vi "AcquireSingleScan.vi"() -> ()   [LabVIEW 2024]
uses:
  X-Scales.ctl
  ff6a1ae8-2aae-4c4f-bccd-18872fa50bd4.vi
  Program Files (x86)/Luna Technologies/OVA 5000 v5.14.2/data/OVA32.dll
panel:
  in  "Num Averages":u32=1
  in  "Output Spreadsheet File Path":path=path "C:/ss.txt"
  in  "Source Matrix":u8(ring) items=["A", "B", "C"]
  in  "Graph Data to Output":bool[](array[boolean])
  in  "Filter?":bool=TRUE
  in  "Resolution BW (GHz)":dbl=5.0 format="%.2f"
  in  "RBW Units for Output":u8(ring) items=["pm", "GHz"]
  in  "Cursor Indices":u32[](array[numeric])=[0, 0]
  in  "Device Descriptor":string
  in  "chanwidthstr":string
  out "error out":errorcluster
  in  "error in (no error)":errorcluster
  in  "Save Data":bool
  in  "Plot Data":bool
  in  "New Scan":bool
  out "Finding DUT Length":bool
  in  "Find DUT Length?":bool
  in  "filter data?":bool
  out "Graph":T1(graph) caption="Insertion Loss"
  in  "X-axis units":T2
  in  "Group Index":dbl=1.5 format="%.2f"
  in  "res BW (GHz)":dbl format="%.2f"
  out "genOutput":dbl[](array[numeric]) format="%.2f"
  in  "Graph Sel":u16(ring) items=["Insertion Loss", "Group Delay", "Chromatic Dispersion", "Polarization Dependent Loss", "Polarization Mode Dispersion", "Linear Phase Deviation", "Quadratic Phase Deviation", "Jones Matrix Element Amplitudes", "Jones Matrix Element Phases", "Time Domain Amplitude", "Time Domain Wavelength", "Min/Max Loss", "Second Order PMD", "Phase Ripple Linear", "Phase Ripple Quadratic"]
  out "error":errorcluster
  in  "Length of DUT (m)":dbl=3.0 format="%.3f"
  in  "Center WL":dbl=1550.0 caption="Center Wavelength (nm)" step=0.01 format="%.2f"
  in  "Meas Type":u16(ring)=1 caption="Type of Measurement" items=["Reflection", "Transmission"]
  in  "WL Range":u16(ring)=2 caption="Wavelength Range (nm)" items=["0.63", "1.27", "2.54", "5.09", "10.22", "20.58", "41.72", "85.78"]
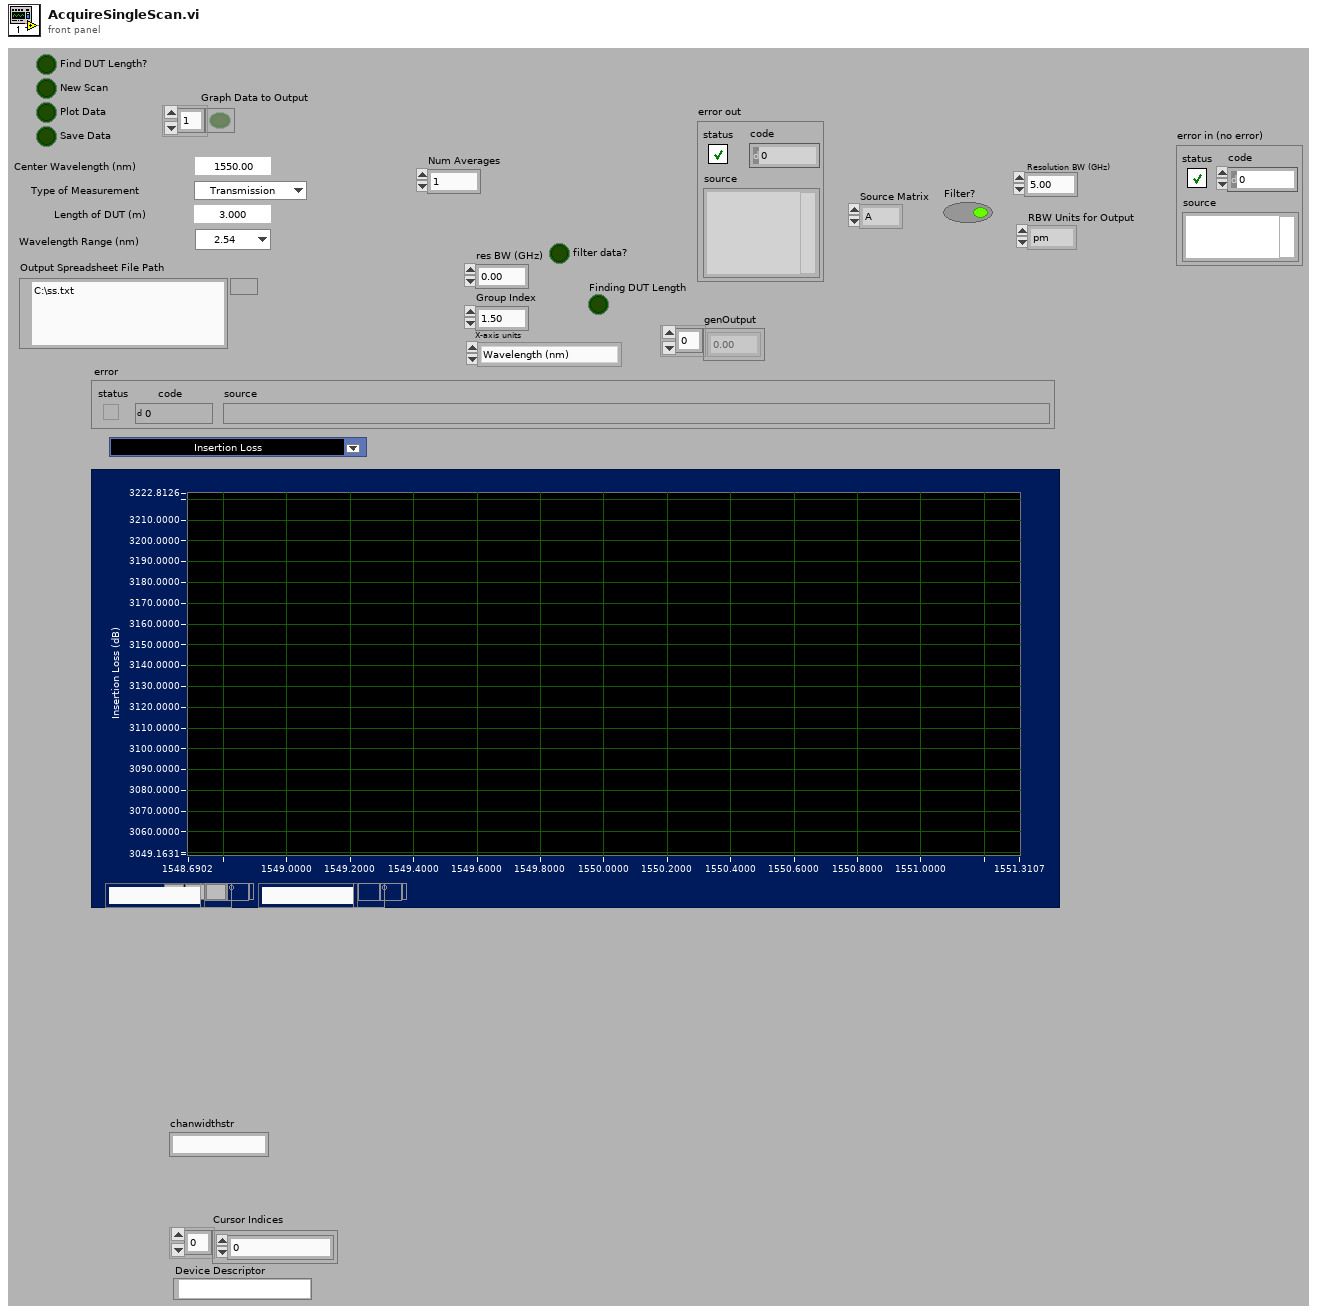
[diagram p1: front panel]
types:
  T1 = cluster{"Array Constant":dbl[], "Array Constant":dbl[]}[]
  T2 = typedef "X-Scales.ctl" = enum16{"Wavelength (nm)", "Gigahertz (GHz)", "Terahertz (THz)", "Time (ns)", "Length (m)"}
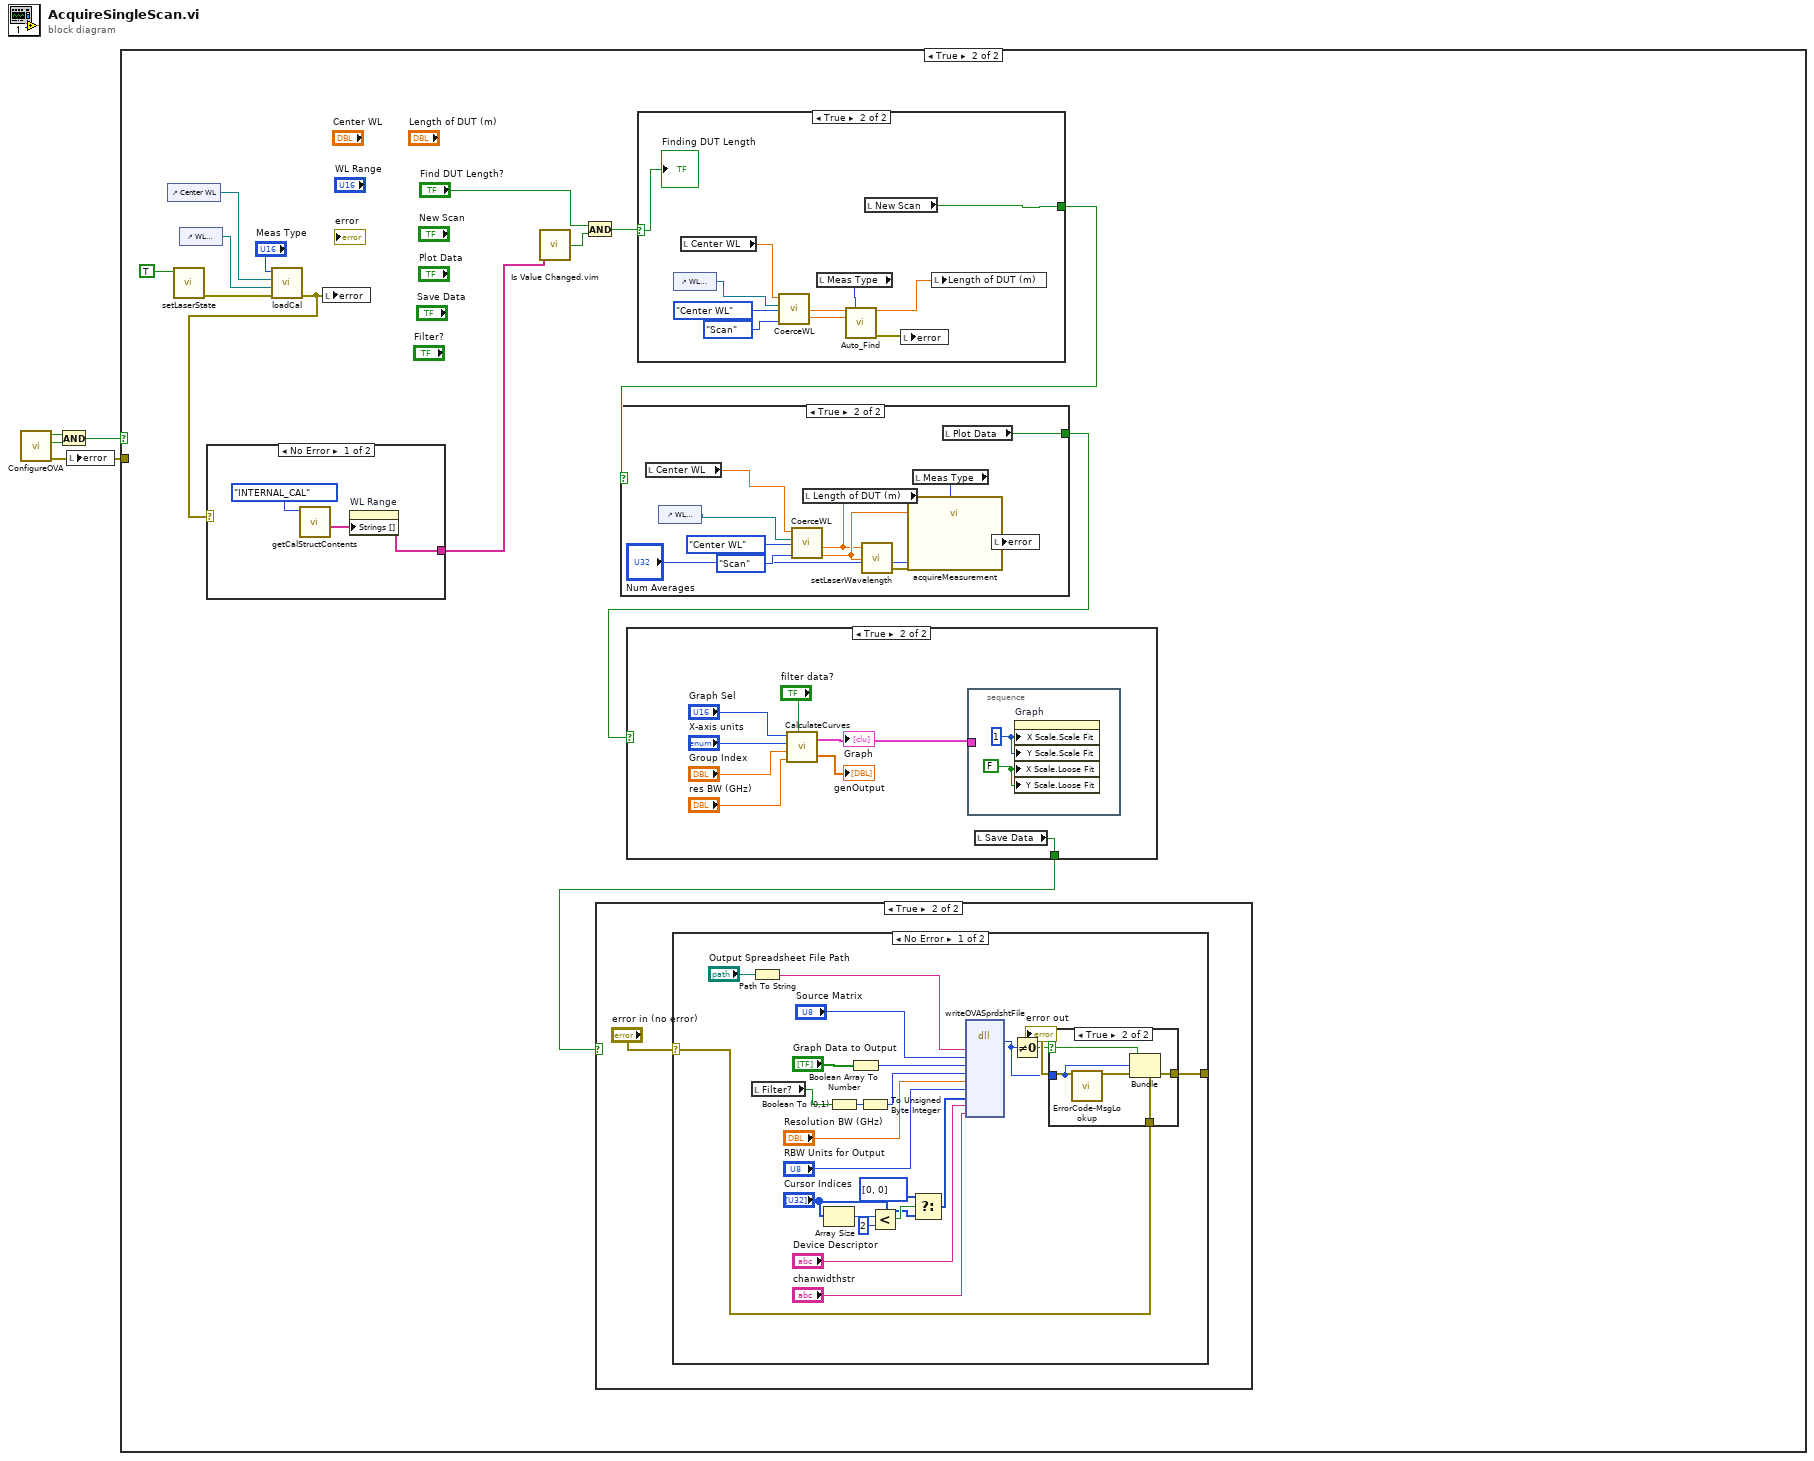
[diagram p0: block diagram]
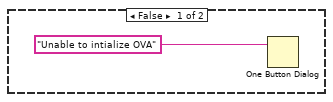
[diagram p2: hidden frame]
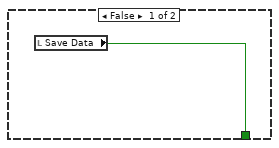
[diagram p6: hidden frame]
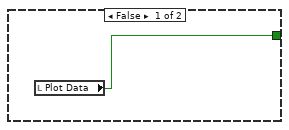
[diagram p7: hidden frame]
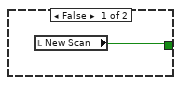
[diagram p8: hidden frame]
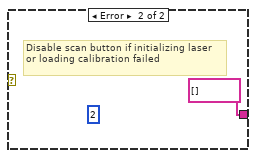
[diagram p9: hidden frame]
diagram:
  n1 = call "ConfigureOVA.vi"() -> ("error out"=w1:errorcluster, "Cfg OK?"=w3:bool, "instrFound"=w4:bool)  [unwired: 4 in, 1 out]
  n2 = And(x=w4, y=w3) -> (x .and. y?=w2:bool)
  n3 = local write "error"(w1) -> ()
  n4 = case shown="True" w2 {
    tunnel: w1 -> [_ _]
    frame False {
      n5 = One Button Dialog(message="Unable to intialize OVA") -> ()  [unwired: 1 in, 1 out]
    }
    frame True {
      n6 = control-ref of="Center WL"() -> (w13:refnum<vi>)
      n7 = call "setLaserState.vi"("New Laser Status"=TRUE) -> ("error out"=w17:errorcluster)  [unwired: 6 in]
      n8 = control-ref of="WL Range"() -> (w15:refnum<vi>)
      n9 = call "loadCal.vi"("error in (no error)"=w17, "Wavelength Range (nm)"=w15, "Center WL (nm)"=w13, "Type of Measurement"="Meas Type") -> ("error out"=w14:errorcluster)  [unwired: 6 in, 1 out]
      n10 = case shown="No Error" w14 {
        tunnel: [w87 string[] [] ("Range Strings")] -> w10
        frame No Error {
          n11 = call "getCalStructContents.vi"("calType"=enum16{"INTERNAL_CAL", "FULL_CAL"}."INTERNAL_CAL" ("Enum")) -> ("Range Strings"=w87:string[])  [unwired: 7 in, 3 out]
          n12 = property on="WL Range" class="Ring (strict)"("Strings []"=w87) -> ()  [unwired: 2 in, 2 out]
        }
        frame Error {
          (unwired) u8 2 ("Disabled")
          # "Disable scan button if initializing laser or loading calibration failed"
        }
      }
      n13 = local write "error"(w14) -> ()
      n14 = call "Is Value Changed.vim"("value"=w10) -> ("changed or first call?"=w9:bool)
      n15 = And(x="Find DUT Length?", y=w9) -> (x .and. y?=w11:bool)
      n16 = case shown="True" w11 {
        selector: w11 -> [_ w85]
        tunnel: [w74 w75] -> w8
        frame False {
          n17 = local read "New Scan"() -> (w74:bool)
        }
        frame True {
          n18 = control-ref of="WL Range"() -> (w83:refnum<vi>)
          n19 = local read "Center WL"() -> (w84:dbl)
          n20 = call "CoerceWL.vi"("Parameter Type"=enum16{"Calibration", "Scan"}."Scan", "wlType"=enum16{"Center WL", "Start WL"}."Center WL", "Wavelength Range (nm)"=w83, "Start/Center Wavelength (nm)"=w84) -> ("end WL (nm)"=w81:dbl, "start WL (nm)"=w80:dbl)  [unwired: 4 in, 2 out]
          n21 = local read "Meas Type"() -> (w79:u16)
          n22 = call "Auto_Find.vi"("Start WL -- nm"=w80, "Type of Measurement"=w79, "End WL -- nm"=w81) -> ("Length of DUT (m)"=w76:dbl, "error out"=w82:errorcluster)  [unwired: 10 in, 1 out]
          n23 = local read "New Scan"() -> (w75:bool)
          n24 = local write "error"(w82) -> ()
          n25 = local write "Length of DUT (m)"(w76) -> ()
          "Finding DUT Length" <- w85
        }
      }
      n26 = case shown="True" w8 {
        tunnel: [w61 w63] -> w7
        frame False {
          n27 = local read "Plot Data"() -> (w61:bool)
        }
        frame True {
          n28 = local read "Center WL"() -> (w71:dbl)
          n29 = control-ref of="WL Range"() -> (w70:refnum<vi>)
          n30 = call "CoerceWL.vi"("Parameter Type"=enum16{"Calibration", "Scan"}."Scan", "wlType"=enum16{"Center WL", "Start WL"}."Center WL", "Wavelength Range (nm)"=w70, "Start/Center Wavelength (nm)"=w71) -> ("end WL (nm)"=w67:dbl, "start WL (nm)"=w66:dbl)  [unwired: 4 in, 2 out]
          n31 = local read "Length of DUT (m)"() -> (w72:dbl)
          n32 = call "setLaserWavelength.vi"("End Wavelength (nm)"=w67, "Start Wavelength (nm)"=w66) -> ("error out"=w68:errorcluster)  [unwired: 2 in, 1 out]
          n33 = local read "Meas Type"() -> (w69:u16)
          n34 = call "acquireMeasurement.vi"("startWL (nm)"=w66, "numScans (1)"="Num Averages", "Type of Measurement"=w69, "endWL (nm)"=w67, "dutLength (m)"=w72, "error in (no error)"=w68) -> ("error out"=w73:errorcluster)  [unwired: 4 in, 5 out]
          n35 = local read "Plot Data"() -> (w63:bool)
          n36 = local write "error"(w73) -> ()
        }
      }
      n37 = case shown="True" w7 {
        tunnel: [w50 w51] -> w6
        frame False {
          n38 = local read "Save Data"() -> (w50:bool)
        }
        frame True {
          n39 = call "CalculateCurves.vi"("Graph Sel"="Graph Sel", "X-axis units"="X-axis units", "Group Index"="Group Index", "res BW (GHz)"="res BW (GHz)", "filter?"="filter data?") -> ("Graph Data"=w52:cluster{dbl[], dbl[]}[], "genOutput"=→"genOutput":dbl[])
          "Graph" <- w52
          n40 = stacked-sequence {
            tunnel: w52 -> [_]
            frame #0 {
              w59 = FALSE ("X Scale.Loose Fit")
              w60 = u8 1 ("X Scale.Scale Fit")
              n41 = property on="Graph" class="XYGraph (strict)"("X Scale.Scale Fit"=w60, "Y Scale.Scale Fit"=w60, "X Scale.Loose Fit"=w59, "Y Scale.Loose Fit"=w59) -> ()  [unwired: 2 in, 2 out]
            }
          }
          n42 = local read "Save Data"() -> (w51:bool)
        }
      }
      n43 = case shown="True" w6 {
        frame False {
        }
        frame True {
          n44 = case shown="No Error" "error in (no error)" {
            selector: "error in (no error)" -> [w32 w49]
            tunnel: [w31 w49] -> w19
            frame No Error {
              n45 = Path To String(path="Output Spreadsheet File Path") -> (string=w41:string)
              n46 = local read "Filter?"() -> (w21:bool)
              n47 = Array Size(array="Cursor Indices") -> (size(s)=w30:i32)
              n48 = Boolean To (0,1)(Boolean=w21) -> (0, 1=w38:i16)
              n49 = Boolean Array To Number(Boolean array="Graph Data to Output") -> (number=w39:u32)
              n50 = To Unsigned Byte Integer(number=w38) -> (unsigned 8bit integer=w37:u8)
              n51 = Less?(x=w30, y=2) -> (x < y?=w27:bool)
              n52 = Select(t=u32[] [0, 0] ("Cursor Indices"), s=w27, f="Cursor Indices") -> (s? t:f=w25:u32[])
              n53 = dll-call lib="C:/Program Files (x86)/Luna Technologies/OVA 5000 v5.14.2/data/OVA32.dll" fn="writeOVASprdshtFile" label="writeOVASprdshtFile()"("SSFileName"=w41, "measMatrix"="Source Matrix", "graphsFlag"=w39, "filter"=w37, "filterRBW"="Resolution BW (GHz)", "outRBWunits"="RBW Units for Output", "indices"=w25, "descriptor"="Device Descriptor", "chanwidthstr"="chanwidthstr") -> (w33:i32)  [unwired: 12 in, 2 out]
              n54 = Not Equal To 0?(x=w33) -> (x != 0?=w34:bool)
              n55 = case shown="True" w34 {
                selector: w34 -> [_ w45]
                tunnel: w33 -> [_ w46]
                tunnel: w32 -> [w43 w48]
                tunnel: [w43 w44] -> w31
                frame False {
                }
                frame True {
                  n56 = call "ErrorCode-MsgLookup.vi"("DLL Return Code"=w46) -> ("Error String"=w47:string)  [unwired: 2 in, 2 out]
                  n57 = Bundle(cluster=w48, "status"=w45, "code"=w46, "source"=w47) -> (w44:errorcluster)
                }
              }
            }
            frame Error {
            }
          }
          "error out" <- w19
        }
      }
    }
  }
